vi "Find All Top Levels on Disk.vi"() -> ()   [LabVIEW 2020]
panel:
  in  "Tab Control":enum32{"Top-level", "Not In Folder", "Strings"}(tab)
  out "Top-level":path[](array[path])
  out "Not in folder":path[](array[path])
  out "Top-Level string":string
  out "Not In Folder string":string
  out "Closing VIs":i32
  out "error out":errorcluster
  out "Total Number of VIs":i32
  out "Checking Callers":i32
  out "Opening VIs":i32
  in  "Directory to search":path=path "C:/Program Files/National Instruments/LabVIEW 8.2/vi.lib/addons/Simulation Interface"
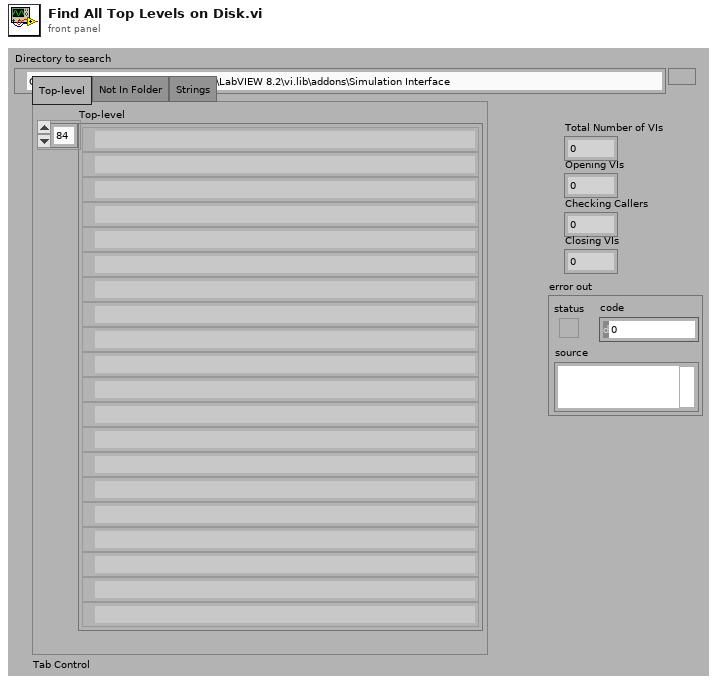
[diagram p1: front panel]
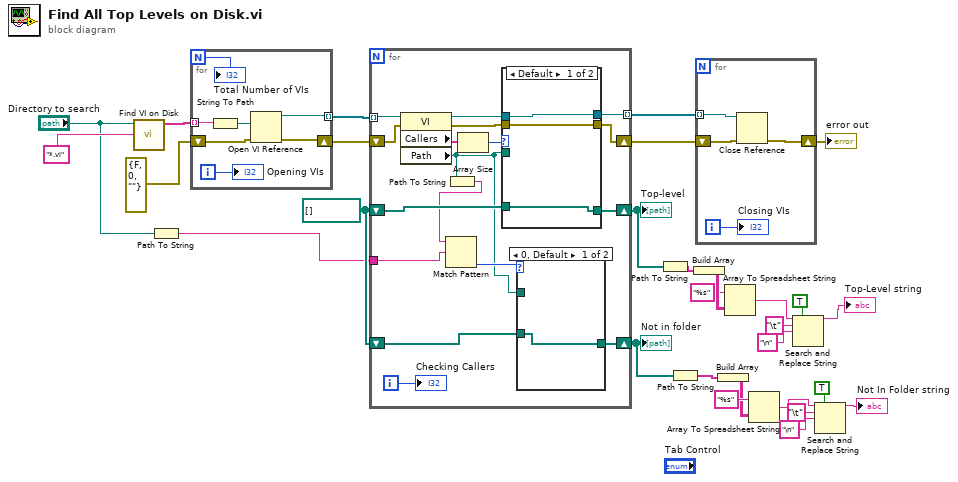
[diagram p0: block diagram]
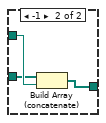
[diagram p2: hidden frame]
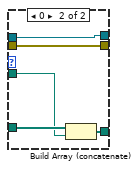
[diagram p3: hidden frame]
diagram:
  w21 = path[] []
  n1 = call "Find VI on Disk.vi"("pattern"="*.vi", "Directory to search"="Directory to search") -> ("Found"=w28:string[])  [unwired: 9 in]
  n2 = Path To String(path="Directory to search") -> (string=w18:string)
  n3 = for {
    N -> [w30]
    tunnel: w28 -> [w36] mode=indexing
    tunnel: [w34] -> w27 mode=indexing
    shift-right: [w33] -> w26
    shift-left: errorcluster {"status"=FALSE, "code"=0, "source"=""} ("error out") -> [w32]
    i -> [w31]
    n4 = String To Path(string=w36) -> (path=w35:path)
    n5 = Open VI Reference(vi path=w35, error in (no error)=w32) -> (vi reference=w34:refnum<vi>, error out=w33:errorcluster)  [unwired: 4 in]
    "Opening VIs" <- w31
    "Total Number of VIs" <- w30
  }
  n6 = for {
    tunnel: w27 -> [w53] mode=indexing
    shift-right: [w47] -> w24
    shift-left: w26 -> [w52]
    tunnel: [w46] -> w25 mode=indexing
    shift-right: [w45] -> w22
    shift-left: w21 -> [w44]
    shift-right: [w39] -> w20
    shift-left: w21 -> [w38]
    tunnel: w18 -> [w37]
    i -> [w43]
    n7 = property class="VI"(reference=w53, error in=w52) -> (reference out=w51:refnum<vi>, error out=w50:errorcluster, "Callers"=w49:string[], "Path"=w40:path)
    n8 = Path To String(path=w40) -> (string=w42:string)
    n9 = Match Pattern(string=w42, regular expression=w37) -> (offset past match=w41:i32)  [unwired: 1 in, 3 out]
    n10 = Array Size(array=w49) -> (size(s)=w48:i32)
    n11 = case shown="Default" w48 {
      tunnel: w51 -> [w59 w62]
      tunnel: w50 -> [w60 w61]
      tunnel: [w60 w61] -> w47
      tunnel: [w59 w62] -> w46
      tunnel: [w58 w65] -> w45
      tunnel: w44 -> [w58 w64]
      tunnel: w40 -> [_ w63]
      frame Default {
      }
      frame 0 {
        n12 = Build Array (concatenate)(w64, w63) -> (w65:path[])
      }
    }
    n13 = case shown="0, Default" w41 {
      tunnel: w40 -> [_ w57]
      tunnel: [w54 w56] -> w39
      tunnel: w38 -> [w54 w55]
      frame 0, Default {
      }
      frame -1 {
        n14 = Build Array (concatenate)(w55, w57) -> (w56:path[])
      }
    }
    "Checking Callers" <- w43
  }
  "Top-level" <- w22
  "Not in folder" <- w20
  n15 = Path To String(path=w22) -> (string=w17:string[])
  n16 = Path To String(path=w20) -> (string=w12:string[])
  n17 = Build Array(w17) -> (w16:string[][])
  n18 = for {
    tunnel: w25 -> [w69] mode=indexing
    shift-right: [w67] -> w23
    shift-left: w24 -> [w68]
    i -> [w66]
    n19 = Close Reference(reference=w69, error in (no error)=w68) -> (error out=w67:errorcluster)
    "Closing VIs" <- w66
  }
  "error out" <- w23
  n20 = Build Array(w12) -> (w13:string[][])
  n21 = Array To Spreadsheet String(array=w16, 3:"%s" ("format string")) -> (spreadsheet string=w7:string)  [unwired: 1 in]
  n22 = Array To Spreadsheet String(array=w13, 3:"%s" ("format string")) -> (spreadsheet string=w2:string)  [unwired: 1 in]
  n23 = Search and Replace String(replace all?=TRUE ("replace all? (F)"), input string=w7, search string="\t", replace string="\n" ("replace string (\"\")")) -> (result string=→"Top-Level string":string)  [unwired: 4 in, 3 out]
  n24 = Search and Replace String(replace all?=TRUE ("replace all? (F)"), input string=w2, search string="\t", replace string="\n" ("replace string (\"\")")) -> (result string=→"Not In Folder string":string)  [unwired: 4 in, 3 out]
